vi "shrink_MM.vi"(8 "Base Values":dbl[](array[numeric]), 9 "pmin_ind":i32, 10 "update M":dbl[][](array[numeric]), 11 "x1":dbl[](array[numeric])) -> (3 "output M":dbl[][](array[numeric]))   [LabVIEW 2015]
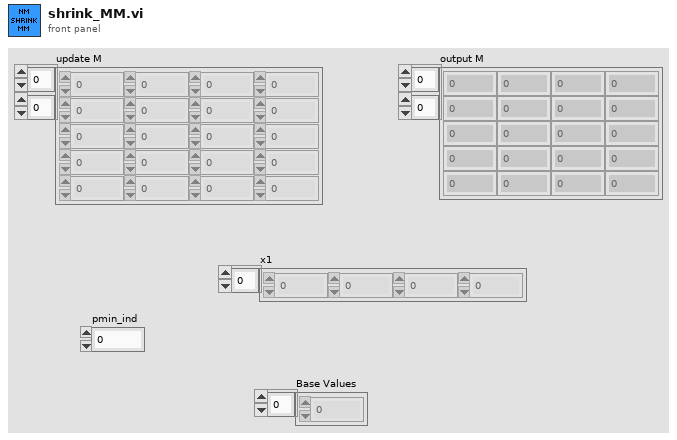
[diagram p1: front panel]
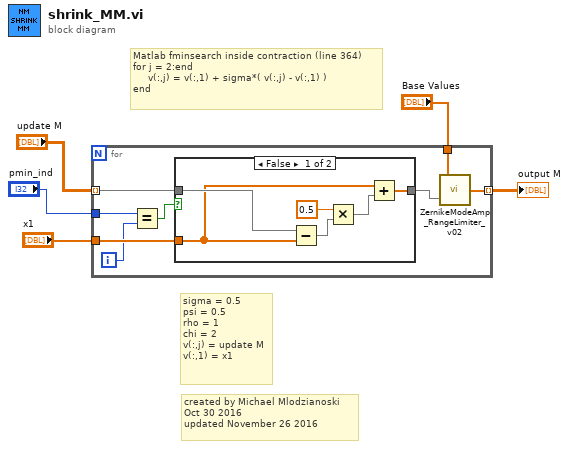
[diagram p0: block diagram]
diagram:
  # "Matlab fminsearch inside contraction (line 364)\nfor j = 2:end\n     v(:,j) = v(:,1) + sigma*( v(:,j) - v(:,1) ) \nend"
  # "created by Michael Mlodzianoski\nOct 30 2016 \nupdated November 26 2016"
  # "sigma = 0.5\npsi = 0.5\nrho = 1\nchi = 2\nv(:,j) = update M\nv(:,1) = x1"
  n1 = for {
    tunnel: "x1" -> [w12]
    tunnel: "update M" -> [w13] mode=indexing
    tunnel: [w7] -> w3 mode=indexing
    tunnel: "pmin_ind" -> [w10]
    tunnel: "Base Values" -> [w6]
    i -> [w11]
    n2 = Equal?(x=w10, y=w11) -> (x = y?=w9:bool)
    n3 = case shown="False" w9 {
      tunnel: w13 -> [w19 w20]
      tunnel: w12 -> [w16 _]
      tunnel: [w14 w20] -> w8
      frame False {
        n4 = Subtract(x=w19, y=w16) -> (x-y=w18:dbl[])
        n5 = Multiply(x=0.5, y=w18) -> (x*y=w15:dbl[])
        n6 = Add(x=w16, y=w15) -> (x+y=w14:dbl[])
      }
      frame True {
      }
    }
    n7 = call "ZernikeModeAmp_RangeLimiter_v02.vi"("x_in"=w8, "Base Values"=w6) -> ("x_out"=w7:dbl[])
  }
  "output M" <- w3
